vi "Reorder variants.vi"(8 "error in (no error)":errorcluster, 10 "Data Variant":variant, 11 "Reference Variant":variant) -> (0 "error out":errorcluster, 3 "Output VData":variant)   [LabVIEW 2015]
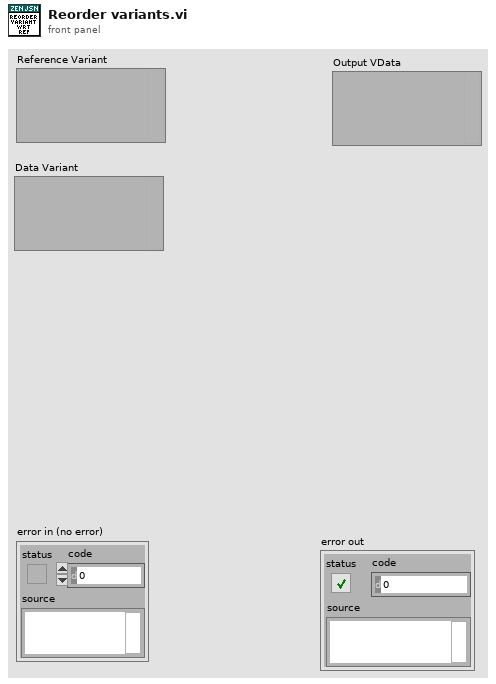
[diagram p1: front panel]
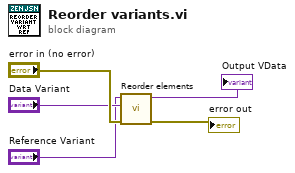
[diagram p0: block diagram]
diagram:
  n1 = call "Reorder elements.vi"("error in (no error)"="error in (no error)", "Data Variant"="Data Variant", "Reference Variant"="Reference Variant") -> ("error out"=→"error out":errorcluster, "Output VData"=→"Output VData":variant)  [unwired: 7 in]
